vi "capstone_main.vi"() -> ()   [LabVIEW 2019]
uses:
  <vilib>/FPGAPlugInAG/myRIO-1900/niLvFpga_Open_myRIO-1900.vi
  <vilib>/rvi/interface/common/dynamic/niFpgaDynamicAddResources.vi
  <vilib>/Utility/error.llb/Error Cluster From Error Code.vi
  <vilib>/rvi/errors/niLvFpgaAdjustHostInterfaceError.vi
  global_stop.vi
  <vilib>/FPGAPlugInAG/Dynamic/niLvFpga_Close_Dynamic.vi
  <vilib>/rvi/interface/nirviOpenFPGA/nirviOpenFPGA.xnode
  FPGA Bitfiles/capstone_FPGATarget_encoderFPGA_AeXAVEDpCcY.lvbitx
  encoder_FPGA.vi
  <vilib>/rvi/interface/nirviReadWriteControl/nirviReadWriteControl.xnode
  <vilib>/rvi/interface/nirviCloseFPGA/nirviCloseFPGA.xnode
  NiFpgaLv.dll
  <vilib>/rvi/interface/Simulation/niFpgaSimulationCallBeginRW.vi
panel:
  out "대포각도":dbl=-50.0
  out "차체회전각도":dbl=-15.552999999999999
  out "-90~90?":bool=TRUE
  out "0~-50":bool
  out "대포를 다 쏘았는가":bool
  in  "wheel_pwm":i32
  in  "정지":bool
  out "i":i32=1583122
  # "FPGA 켜고 와라"
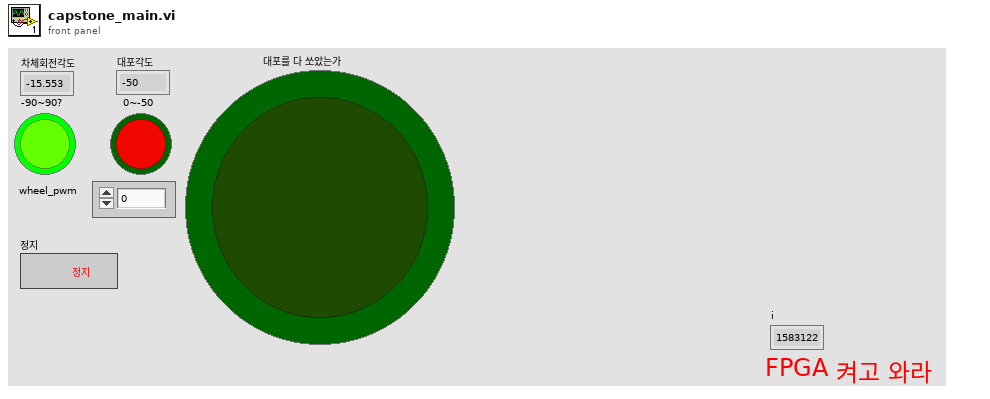
[diagram p1: front panel]
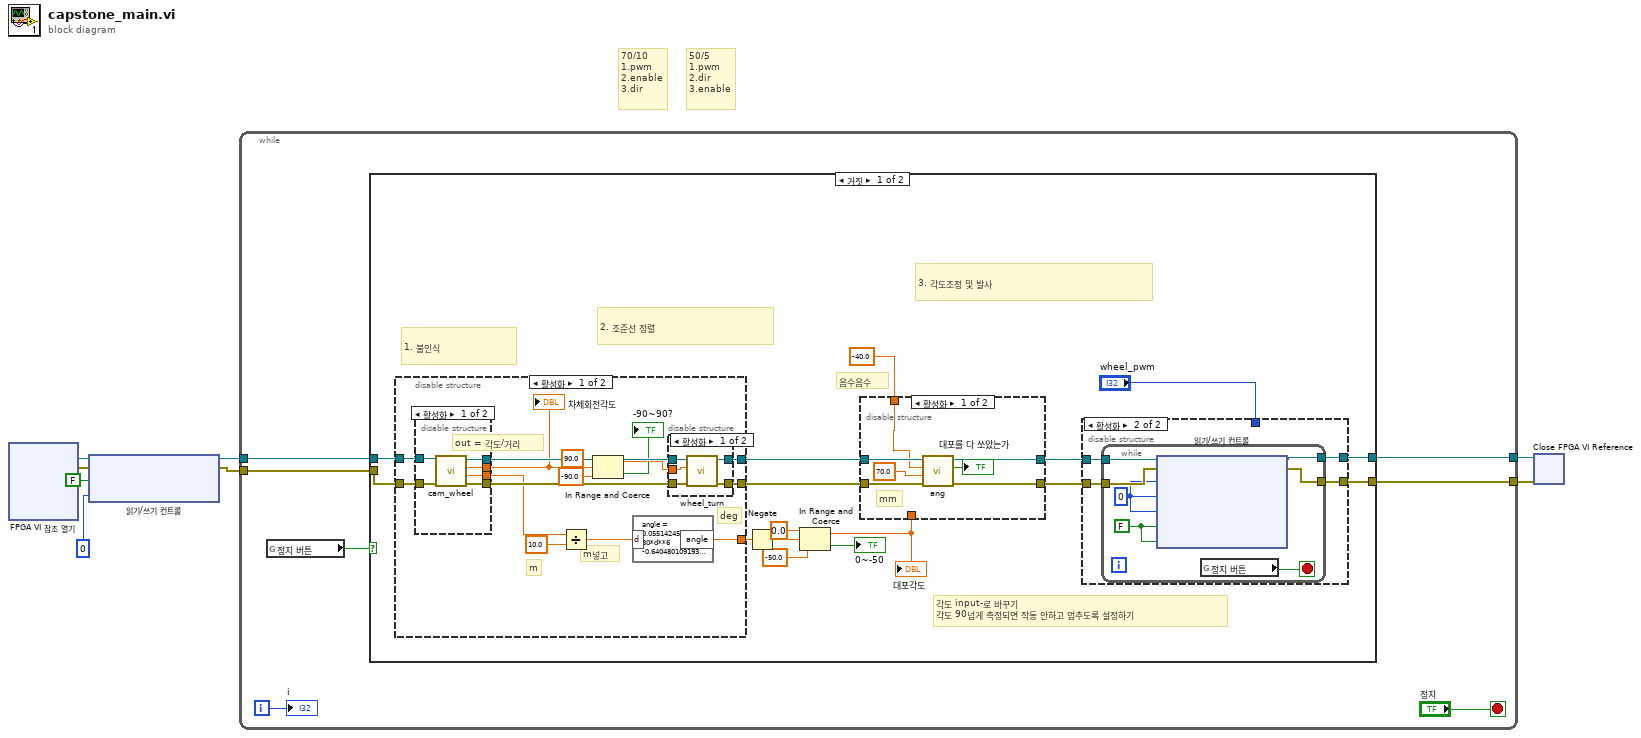
[diagram p0: block diagram]
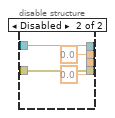
[diagram p4: hidden frame]
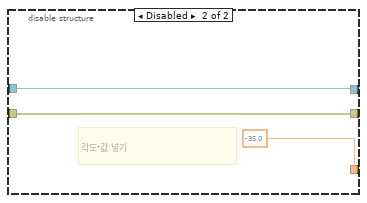
[diagram p5: hidden frame]
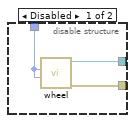
[diagram p6: hidden frame]
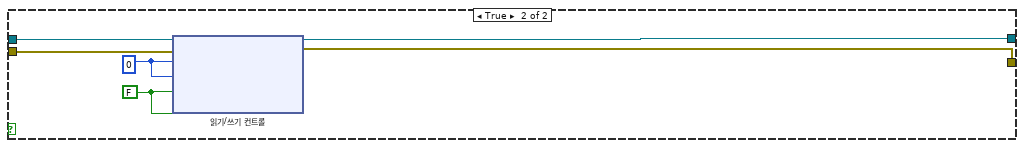
[diagram p7: hidden frame]
diagram:
  # "50/5\n1.pwm\n2.dir\n3.enable"
  # "70/10\n1.pwm\n2.enable\n3.dir"
  n1 = xnode "FPGA VI 참조 열기"() -> ("FPGA VI 참조 출력"=w5:refnum<k20>, "에러 출력"=w2:errorcluster)  [unwired: 2 in]
  n2 = xnode "읽기/쓰기 컨트롤"("FPGA VI 참조 입력"=w5, "에러 입력"=w2, "angle_Enable (escon)"=FALSE, "직동_pwm input"=0) -> ("FPGA VI 참조 출력"=w4:refnum<k20>, "에러 출력"=w3:errorcluster)
  n3 = while {
    tunnel: w4 -> [w10]
    tunnel: w3 -> [w9]
    tunnel: [w12] -> w8
    tunnel: [w11] -> w7
    i -> [w15]
    stop <- "정지" stop-if-true
    n4 = global read "global_stop.vi" "정지 버튼"() -> (w13:bool)
    n5 = case shown="거짓" w13 {
      tunnel: w10 -> [w31 w93]
      tunnel: w9 -> [w30 w92]
      tunnel: [w23 w95] -> w12
      tunnel: [w22 w94] -> w11
      frame False {
        # "2. 조준선 정렬"
        # "3. 각도조정 및 발사"
        # "1. 불인식"
        # "음수음수"
        # "각도 input-로 바꾸기\n각도 90넘게 측정되면 작동 안하고 멈추도록 설정하기"
        n6 = disable-structure shown="활성화" {
          disable-tunnel: w31 -> [w55 w75]
          disable-tunnel: w30 -> [w54 w74]
          disable-tunnel: [w52 w75] -> w21
          disable-tunnel: [w51 w74] -> w20
          disable-tunnel: [w49 -35.0 ("wanted angle")] -> w25
          frame Enabled {
            # "m"
            # "deg"
            # "m넣고"
            # "out = 각도/거리"
            n7 = disable-structure shown="활성화" {
              disable-tunnel: w55 -> [w68 w72]
              disable-tunnel: w54 -> [w67 w71]
              disable-tunnel: [w66 w72] -> w53
              disable-tunnel: [w65 w71] -> w50
              disable-tunnel: [w64 0.0 ("차체회전각도")] -> w42
              disable-tunnel: [w63 0.0 ("거리")] -> w45
              frame Enabled {
                n8 = call "cam_wheel.vi"("에러 입력"=w67, "FPGA VI 참조 입력"=w68) -> ("에러 출력"=w65:errorcluster, "거리"=w63:dbl, "차체각도"=w64:dbl, "FPGA VI 참조 출력"=w66:refnum<k20>)  [unwired: 5 in]
              }
              frame Disabled {
              }
            }
            "차체회전각도" <- w42
            n9 = Divide(x=w45, y=10.0) -> (x/y=w44:dbl)
            n10 = In Range and Coerce(upper limit=90.0 ("상위 리미트"), x=w42, lower limit=-90.0 ("하위 리미트")) -> (coerced(x)=w41:dbl, In Range?=→"-90~90?":bool)
            n11 = formula code="angle = 0.0551424574910630*d**6       -0.640480109193604*d**5       +2.83568223661573*d**4     -5.78893038911684*d**3     +5.55222793824200*d**2       +4.45825307955888*d**1         +0.151173722799724*d**0;"("d"=w44) -> ("angle"=w49:dbl)
            n12 = disable-structure shown="활성화" {
              disable-tunnel: w53 -> [w60 w62]
              disable-tunnel: [w59 w62] -> w52
              disable-tunnel: [w58 w61] -> w51
              disable-tunnel: w50 -> [w57 w61]
              disable-tunnel: w41 -> [w56 _]
              frame Enabled {
                n13 = call "wheel_turn.vi"("에러 입력"=w57, "wanted angle(deg)"=w56, "FPGA VI 참조 입력"=w60) -> ("에러 출력"=w58:errorcluster, "FPGA VI 참조 출력"=w59:refnum<k20>)  [unwired: 7 in]
              }
              frame Disabled {
              }
            }
          }
          frame Disabled {
            # "각도-값 넣기"
          }
        }
        n14 = Negate(x=w25) -> (-x=w24:dbl)
        n15 = In Range and Coerce(upper limit=0.0 ("상위 리미트"), x=w24, lower limit=-50.0 ("하위 리미트")) -> (coerced(x)=w17:dbl, In Range?=→"0~-50":bool)
        "대포각도" <- w17
        n16 = disable-structure shown="활성화" {
          disable-tunnel: w21 -> [w38 w40]
          disable-tunnel: w20 -> [w37 w39]
          disable-tunnel: [w36 w40] -> w19
          disable-tunnel: [w35 w39] -> w18
          disable-tunnel: w17 -> [_ _]
          disable-tunnel: -40.0 ("wanted angle") -> [w32 _]
          frame Enabled {
            # "mm"
            n17 = call "ang.vi"("에러 입력"=w37, "spring pull"=70.0, "wanted angle"=w32, "FPGA VI 참조 입력"=w38) -> ("에러 출력"=w35:errorcluster, "대포를 다 쏨????"=→"대포를 다 쏘았는가":bool, "FPGA VI 참조 출력"=w36:refnum<k20>)  [unwired: 5 in]
          }
          frame Disabled {
          }
        }
        n18 = disable-structure shown="활성화" {
          disable-tunnel: [w78 w80] -> w23
          disable-tunnel: [w77 w79] -> w22
          disable-tunnel: w19 -> [_ w82]
          disable-tunnel: w18 -> [_ w81]
          disable-tunnel: "wheel_pwm" -> [w76 _]
          frame Disabled {
            n19 = call "wheel.vi"("R_pwm"=w76, "L_pwm"=w76) -> ("에러 출력"=w77:errorcluster, "FPGA VI 참조 출력"=w78:refnum<k20>)  [unwired: 8 in]
          }
          frame Enabled {
            n20 = while {
              tunnel: w82 -> [w89]
              tunnel: w81 -> [w88]
              tunnel: [w87] -> w80
              tunnel: [w86] -> w79
              stop <- w83 stop-if-true
              w84 = 0 ("pwm input")
              w85 = FALSE ("angle_Enable (escon)")
              n21 = xnode "읽기/쓰기 컨트롤"("FPGA VI 참조 입력"=w89, "에러 입력"=w88, "pwm input"=w84, "R_pwm input"=w84, "직동_pwm input"=w84, "angle_Enable (escon)"=w85, "tir_Enable (escon)"=w85) -> ("FPGA VI 참조 출력"=w87:refnum<k20>, "에러 출력"=w86:errorcluster)
              n22 = global read "global_stop.vi" "정지 버튼"() -> (w83:bool)
            }
          }
        }
      }
      frame True {
        w91 = FALSE ("angle_Enable (escon)")
        w90 = 0 ("직동_pwm input")
        n23 = xnode "읽기/쓰기 컨트롤"("FPGA VI 참조 입력"=w93, "에러 입력"=w92, "직동_pwm input"=w90, "pwm input"=w90, "angle_Enable (escon)"=w91, "tir_Enable (escon)"=w91) -> ("FPGA VI 참조 출력"=w95:refnum<k20>, "에러 출력"=w94:errorcluster)
      }
    }
    "i" <- w15
  }
  n24 = xnode "Close FPGA VI Reference"("FPGA VI 참조 입력"=w8, "에러 입력"=w7) -> ()  [unwired: 1 out]
